vi "GenerateLogFilePath.vi"(8 "error in (no error)":errorcluster) -> (0 "error out":errorcluster, 3 "actual path":path)   [LabVIEW 2019, in "Log.Litho.lvclass"]
uses:
  Log.Litho.lvclass
  <vilib>/Utility/sysdir.llb/Get System Directory.vi
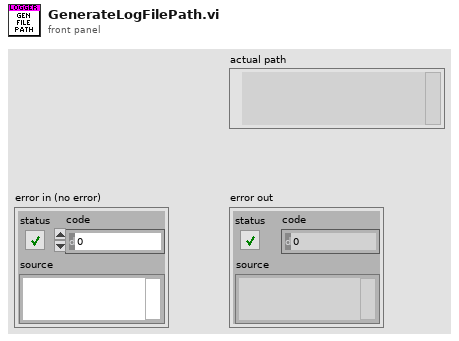
[diagram p1: front panel]
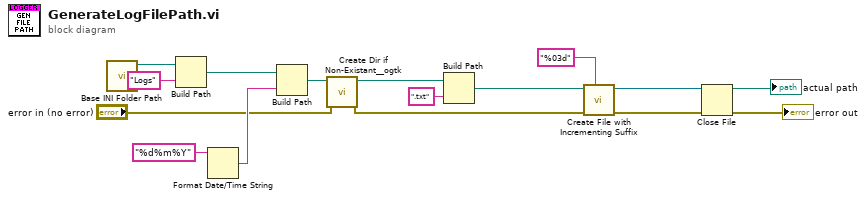
[diagram p0: block diagram]
diagram:
  n1 = call "Base INI Folder Path.vi"() -> ("Base Path"=w12:path)  [unwired: 11 in]
  n2 = Build Path(base path=w12, name or relative path="Logs") -> (appended path=w13:path)
  n3 = Format Date/Time String(time format string (%c)="%d%m%Y") -> (date/time string=w14:string)  [unwired: 2 in]
  n4 = Build Path(base path=w13, name or relative path=w14) -> (appended path=w15:path)
  n5 = call <userlib>:"Create Dir if Non-Existant__ogtk.vi"("error in (no error)"="error in (no error)", "Directory Path"=w15) -> ("error out"=w4:errorcluster, "dup Directory Path"=w16:path)  [unwired: 7 in, 1 out]
  n6 = Build Path(base path=w16, name or relative path=".txt") -> (appended path=w8:path)
  n7 = call <vilib>:"Create File with Incrementing Suffix.vi"("format string (\" (%d)\")"="%03d" ("format string (\" (%d)\")"), "error in (no error)"=w4, "file path"=w8) -> ("error out"=w5:errorcluster, "refnum out"=w7:refnum<file>)  [unwired: 6 in, 1 out]
  n8 = Close File(refnum=w7, error in=w5) -> (path=→"actual path":path, error out=→"error out":errorcluster)
